vi "ImageInit.vi"(0 "Image in":refnum<class "Image.lvclass">, 1 "Stage Acquire Parameters":T3={"Scan Mode"=enum."Continuous", "Start position mm"=115.0, "End position mm"=112.0, "Velocity um/sec (continuous)"=200.0, "Step size microns (discrete)"=0.0, "Frames to grab (grab)"=200} {"End position mm" format="%_6g"; "Start position mm" format="%_6g"}, 2 "Hardware Settings":T1={"Galvo Channels"="Dev1/ao0:1", "Detector Channels"="Dev1/ai0:2", "Galvo Trigger"="/Dev1/ai/StartTrigger", "Shutter Lines"=["Dev1/port0/line7"], "Max Acquisition Rate"=5000000.0, "Recommended Acquisition Rate"=5000000.0, "Galvo Write Rate"=2500000.0, "Max Timebase Frequency (Hz)"=20000000.0, "MCC Shutter Lines"=[], "Detector Task"="", "Shutter Tasks"=[], "Galvo Task"="", "Digital Image Multiplier"=[100.0, 100.0, -100.0]} {"Max Acquisition Rate" min=0.0 max=5000000.0 step=100000.0}, 3 "Scan Parameters":T2={"x pixels"=256, "x voltage min"=-2.0, "x voltage max"=2.0, "y voltage min"=256.0, "y voltage max"=-2.0, "fill frac"=2.0, "Zoom"=1.0, "BiDi"=FALSE, "scan rate (ms/line)"=2.0} {"Zoom" min=0.0 max=1.0 step=1.0; "fill frac" format="%0.2p"; "y voltage max" format="%0.2p"; "x voltage max" format="%0.2p"; "x voltage min" format="%0.2p"}, 5 "Save Path":path=path "C:/Users/Jeremy/Desktop", 9 "Filename":string="test", 11 "error in (no error)":errorcluster, 12 "show flyback data":bool, 13 "disable averaging":bool, 14 "Autosave":bool) -> (4 "Image out":refnum<class "Image.lvclass">, 15 "error out":errorcluster)   [LabVIEW 2012, in "Image.lvclass"]
uses:
  classes/Image.lvclass
  typedefs/Stage Parameters.ctl
  typedefs/ScanMode.ctl
  typedefs/Scan Parameters.ctl
  typedefs/HWsettings.ctl
  classes/Image.lvclass/Image.ctl
  typedefs/DetectorType.ctl
  <resource>/objmgr/daqmx.rc
panel:
  out "NumChans":u32
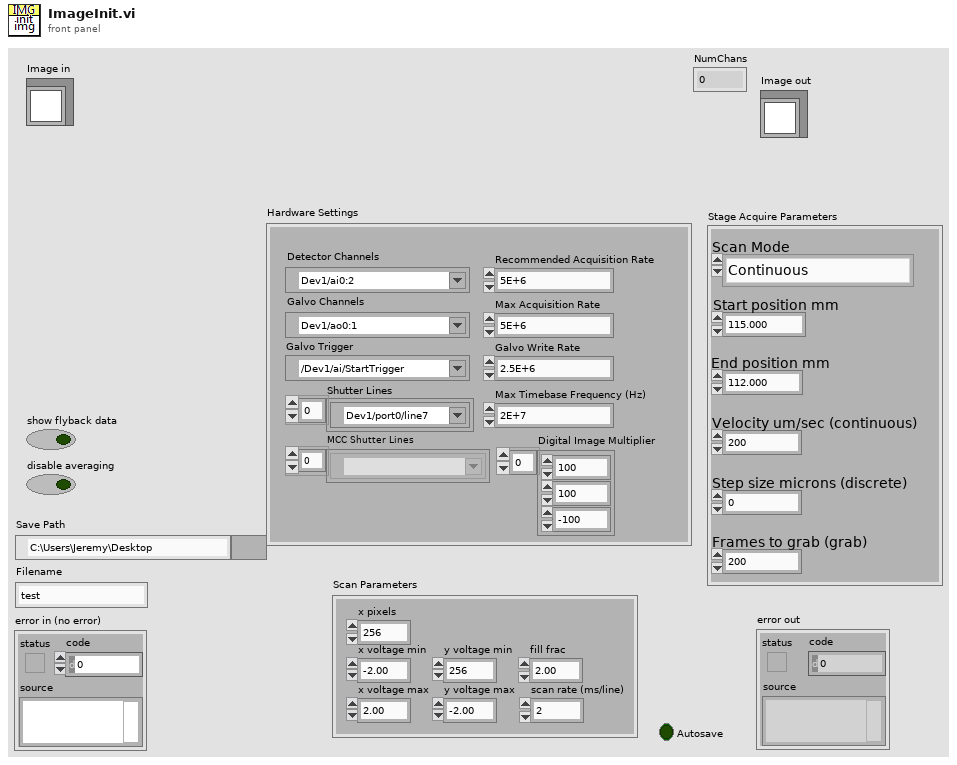
[diagram p1: front panel]
types:
  T1 = typedef "HWsettings.ctl" = cluster{"Galvo Channels":tag, "Detector Channels":tag, "Galvo Trigger":tag, "Shutter Lines":tag[], "Max Acquisition Rate":dbl, "Recommended Acquisition Rate":dbl, "Galvo Write Rate":dbl, "Max Timebase Frequency (Hz)":dbl, "MCC Shutter Lines":refnum<k21>[], "Detector Task":refnum<k21>, "Shutter Tasks":refnum<k21>[], "Galvo Task":refnum<k21>, "Digital Image Multiplier":dbl[]}
  T2 = typedef "Scan Parameters.ctl" = cluster{"x pixels":i32, "x voltage min":dbl, "x voltage max":dbl, "y voltage min":dbl, "y voltage max":dbl, "fill frac":dbl, "Zoom":dbl, "BiDi":bool, "scan rate (ms/line)":dbl}
  T3 = typedef "Stage Parameters.ctl" = cluster{"Scan Mode":T4, "Start position mm":dbl, "End position mm":dbl, "Velocity um/sec (continuous)":dbl, "Step size microns (discrete)":dbl, "Frames to grab (grab)":i32}
  T4 = typedef "ScanMode.ctl" = enum16{"None", "Continuous", "Point Scan (CH3 cursor)", "Point Scan Move (CH3 cursor)", "Grab", "Grab Move Stage", "Grab Move Z-stage", "Cont. Move Z-stage", "Spec Move Stage", "Spec Move Cont", "Surf Calib"}
  T5 = typedef "DetectorType.ctl" = enum16{"PMT", "SpectraWiz"}
  T6 = typedef "ScanModeScanType.ctl" = enum16{"default", "point scan", "grab"}
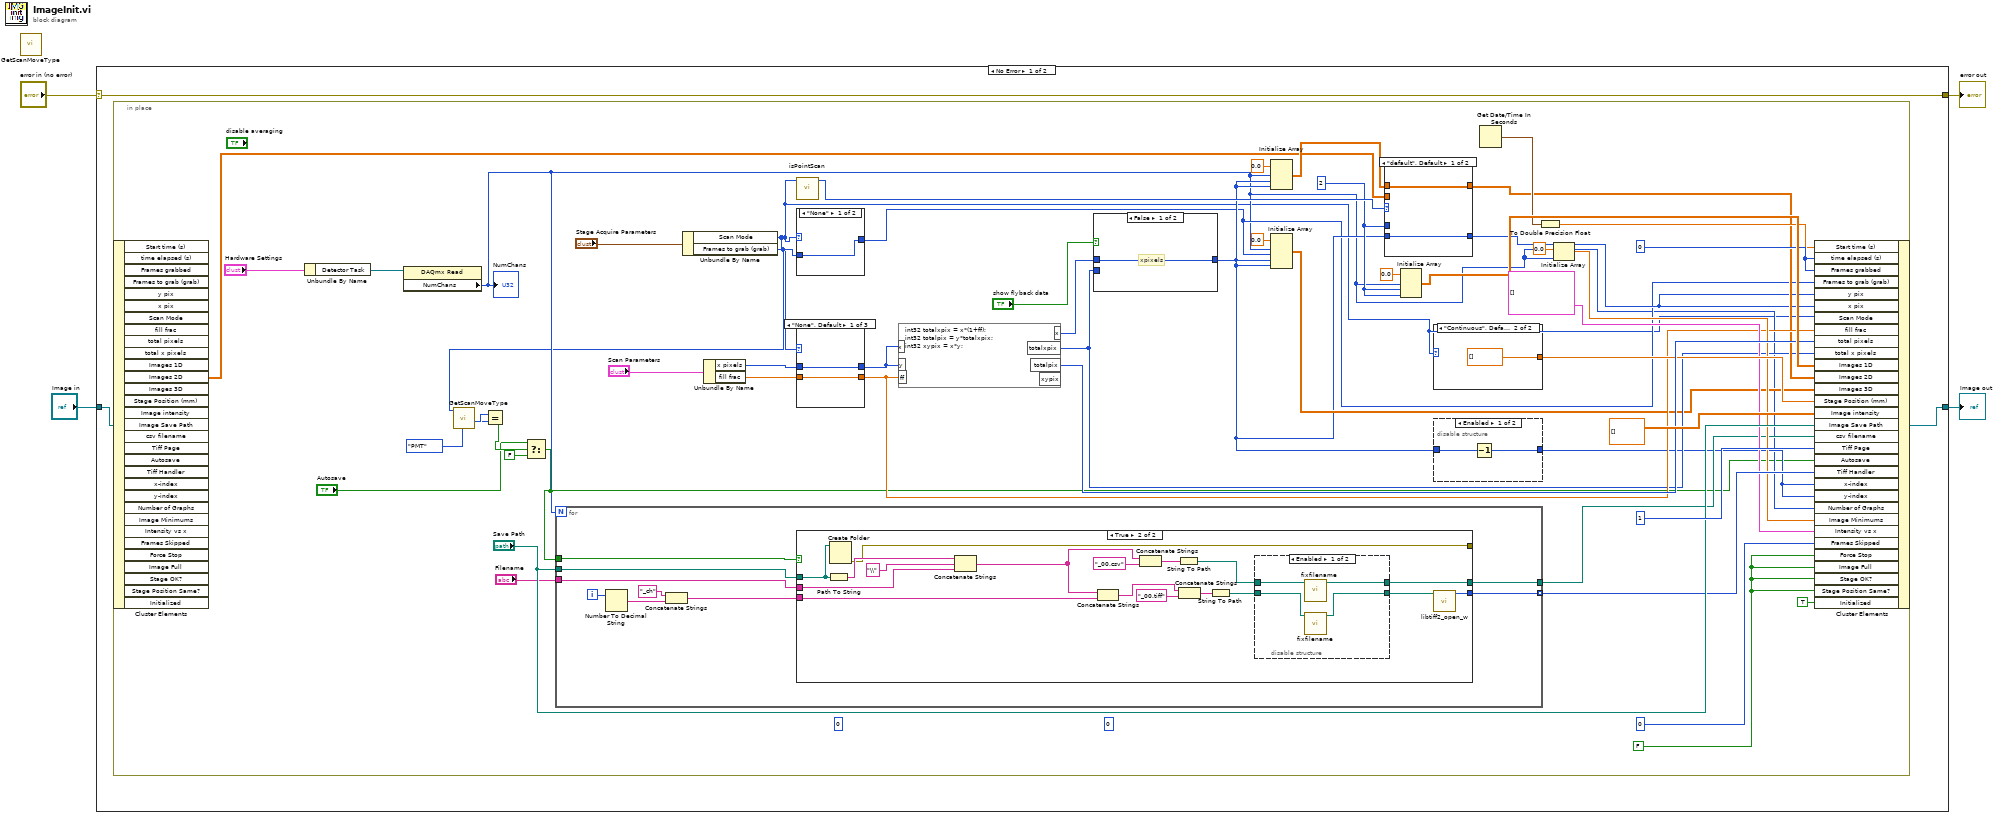
[diagram p0: block diagram]
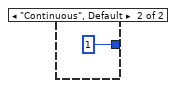
[diagram p2: hidden frame]
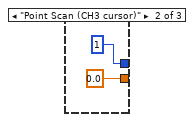
[diagram p5: hidden frame]
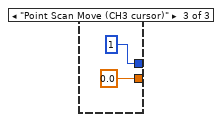
[diagram p6: hidden frame]
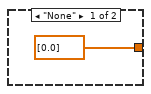
[diagram p10: hidden frame]
diagram:
  n1 = call "GetScanMoveType.vi"() -> ()  [unwired: 9 in, 3 out]
  n2 = case shown="No Error" "error in (no error)" {
    selector: "error in (no error)" -> [w7 w111]
    tunnel: [w7 w111] -> w3
    tunnel: [w5 w110] -> w1
    tunnel: "Image in" -> [w6 w110]
    frame No Error {
      n3 = in-place {
        w25 = 2 ("dimension size")
        w24 = FALSE ("Force Stop")
        w42 = 0 ("Frames grabbed")
        (unwired) 0 ("y-index")
        (unwired) 0 ("x-index")
        n4 = in-place-cluster #1(w6) -> ("Images 2D"=w28:dbl[][][])  [unwired: 30 out]
        n5 = Unbundle By Name("Hardware Settings") -> ("Detector Task"=w48:refnum<k21>)
        n6 = property class="DAQmx Read"(reference=w48) -> ("NumChans"=w16:u32)  [unwired: 1 in, 2 out]
        "NumChans" <- w16
        n7 = Unbundle By Name("Stage Acquire Parameters") -> ("Scan Mode"=w14:T4, "Frames to grab (grab)"=w18:i32)
        n8 = call "GetScanMoveType.vi"("Scan Mode"=w14) -> ("Detector"=w13:T5)  [unwired: 8 in, 2 out]
        n9 = Equal?(x=w13, y=DetectorType."PMT" ("Detector")) -> (x = y?=w11:bool)
        n10 = Select(t="Autosave", s=w11, f=FALSE) -> (s? t:f=w8:bool)
        n11 = for {
          N: w16 -> [_]
          tunnel: "Filename" -> [w76]
          tunnel: w8 -> [w84]
          tunnel: "Save Path" -> [w82]
          tunnel: [w81] -> w49 mode=indexing
          tunnel: [w77] -> w38
          i -> [w80]
          n12 = Number To Decimal String(number=w80) -> (decimal integer string=w79:string)  [unwired: 1 in]
          n13 = Concatenate Strings("_ch" ("string"), w79) -> (w83:string)
          n14 = case shown="True" w84 {
            tunnel: w83 -> [_ w93]
            tunnel: w82 -> [_ w86]
            tunnel: [_ w99] -> w81
            tunnel: [_ w88] -> w77
            tunnel: w76 -> [_ w94]
            tunnel: [_ w85] -> _
            frame False {
            }
            frame True {
              n15 = Path To String(path=w86) -> (string=w100:string)
              n16 = Create Folder(path (use dialog)=w86) -> (error out=w85:errorcluster)  [unwired: 2 in, 2 out]
              n17 = Concatenate Strings(w100, "\\" ("string"), w94) -> (w91:string)
              n18 = Concatenate Strings(w91, w93) -> (w92:string)
              n19 = Concatenate Strings(w91, "_00.csv" ("string")) -> (w95:string)
              n20 = String To Path(string=w95) -> (path=w89:path)
              n21 = Concatenate Strings(w92, "_00.tiff" ("string")) -> (w97:string)
              n22 = String To Path(string=w97) -> (path=w90:path)
              n23 = disable-structure shown="Enabled" {
                disable-tunnel: w90 -> [w105 w106]
                disable-tunnel: w89 -> [w104 w107]
                disable-tunnel: [w103 w107] -> w88
                disable-tunnel: [w102 w106] -> w87
                frame Enabled {
                  n24 = call "fixfilename.vi"("Path"=w104) -> ("fixed path"=w103:path)  [unwired: 9 in, 1 out]
                  n25 = call "fixfilename.vi"("Path"=w105) -> ("fixed path"=w102:path)  [unwired: 9 in, 1 out]
                }
                frame Disabled {
                }
              }
              n26 = call "libtiff2_open_w.vi"("Input path"=w87) -> ("handle"=w99:i32)  [unwired: 9 in, 1 out]
            }
          }
        }
        n27 = Unbundle By Name("Scan Parameters") -> ("x pixels"=w36:i32, "fill frac"=w33:dbl)
        n28 = call "isPointScan.vi"("Scan Mode"=w14) -> ("Scan Type"=w31:T6)  [unwired: 8 in]
        n29 = case shown="\"None\"" w14 {
          tunnel: w18 -> [w59 _]
          tunnel: [w59 1 ("Frames grabbed")] -> w17
          frame "None" {
          }
          frame "Continuous", Default {
          }
        }
        n30 = case shown="\"None\", Default" w14 {
          tunnel: w36 -> [w69 _ _]
          tunnel: [w69 1 1] -> w35
          tunnel: [w68 0.0 ("fill frac") 0.0 ("fill frac")] -> w34
          tunnel: w33 -> [w68 _ _]
          frame "None", Default {
          }
          frame "Point Scan (CH3 cursor)" {
          }
          frame "Point Scan Move (CH3 cursor)" {
          }
        }
        n31 = formula code="int32 totalxpix = x*(1+ff);\nint32 totalpix = y*totalxpix;\nint32 xypix = x*y;"("x"=w35, "y"=w35, "ff"=w34) -> ("totalpix"=w52:i32, "totalxpix"=w27:i32, "x"=w32:i32)  [unwired: 1 out]
        n32 = case shown="False" "show flyback data" {
          tunnel: w27 -> [_ w75]
          tunnel: [w74 w75] -> w20
          tunnel: w32 -> [w74 _]
          frame False {
            # "xpixels"
          }
          frame True {
            # "total x pixels"
          }
        }
        n33 = Initialize Array(0.0 ("element"), w16, w20, w20) -> (w30:dbl[][][])
        n34 = Initialize Array(0.0 ("element"), w16, w17, w20, w20) -> (w22:dbl[][][][])
        n35 = case shown="\"default\", Default" w31 {
          tunnel: w30 -> [w65 _]
          tunnel: [w65 w67] -> w29
          tunnel: w28 -> [_ w67]
          tunnel: [w64 w66] -> w26
          tunnel: w25 -> [_ w66]
          tunnel: w20 -> [w64 _]
          frame "default", Default {
          }
          frame "point scan" {
          }
        }
        n36 = Initialize Array(0.0 ("element"), w16, w25, w25) -> (w53:dbl[][][])
        n37 = case shown="\"Continuous\", Default" w14 {
          tunnel: [dbl[] [0.0] ("Stage Position (mm)") dbl[] [] ("Stage Position (mm)")] -> w51
          frame "None" {
          }
          frame "Continuous", Default {
          }
        }
        n38 = disable-structure shown="Enabled" {
          disable-tunnel: w20 -> [w62 w63]
          disable-tunnel: [w61 w63] -> w19
          frame Enabled {
            n39 = Decrement(x=w62) -> (x-1=w61:i32)
          }
          frame Disabled {
          }
        }
        n40 = Get Date/Time In Seconds() -> (seconds since 1Jan1904=w41:timestamp)
        n41 = To Double Precision Float(number=w41) -> (double precision float=w40:dbl)
        n42 = Initialize Array(0.0 ("element"), w16) -> (w44:dbl[])
        n43 = in-place-cluster #1("Start time (s)"=w40, "time elapsed (s)"=w42, "Frames grabbed"=w42, "Frames to grab (grab)"=w17, "y pix"=w26, "x pix"=w26, "Scan Mode"=w14, "fill frac"=w34, "total pixels"=w52, "total x pixels"=w27, "Images 1D"=w53, "Images 2D"=w29, "Images 3D"=w22, "Stage Position (mm)"=w51, "Image intensity"=dbl[][] [], "Image Save Path"="Save Path", "csv filename"=w38, "Tiff Page"=u32 1, "Autosave"=w8, "Tiff Handler"=w49, "x-index"=w19, "y-index"=w19, "Number of Graphs"=w16, "Image Minimums"=w44, "Intensity vs x"=cluster{dbl[], dbl[]}[] [], "Frames Skipped"=0, "Force Stop"=w24, "Image Full"=w24, "Stage OK?"=w24, "Stage Position Same?"=w24, "Initialized"=TRUE) -> (w5:refnum<class "Image.lvclass">)
      }
    }
    frame Error {
    }
  }
  "error out" <- w3
  "Image out" <- w1
